vi "Custom Assertion Failure Message.vi"() -> ()   [LabVIEW 2017, in "Transparent Assertions.Tests.lvlib" / "Assert Not Error.lvlib"]
uses:
  Assert Not Error.lvlib
  <vilib>/Utility/error.llb/Error Cluster From Error Code.vi
  <vilib>/ErrorRing/Error Ring.xnode
  src/Transparent Assertions/Transparent Assertions.lvlib
panel:
  out "error out":errorcluster
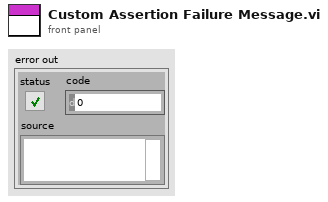
[diagram p1: front panel]
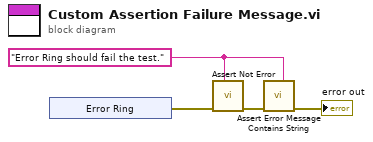
[diagram p0: block diagram]
diagram:
  w1 = "Error Ring should fail the test." ("Message (\"\")")
  n1 = xnode "Error Ring"() -> ("error out"=w4:errorcluster)
  n2 = call "Assert Not Error.vi"("Message (\"\")"=w1, "error in (no error)"=w4) -> ("error out"=w3:errorcluster)  [unwired: 9 in]
  n3 = call "Assert Error Message Contains String.vi"("Expected"=w1, "error in (no error)"=w3) -> ("error out"=→"error out":errorcluster)  [unwired: 9 in]
